vi "d1000 set pls outmode.vi"(10 "pls_outmode":i16, 11 "axis":i16) -> (3 "function return":u32)   [LabVIEW 2019, in "Dmc1000.lvlib"]
doc: "DMC1000_API DWORD WINAPI d1000_set_pls_outmode(short axis,short pls_outmode);"
uses:
  Dmc1000.lvlib
  Dmc1000.dll
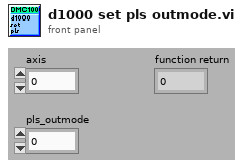
[diagram p1: front panel]
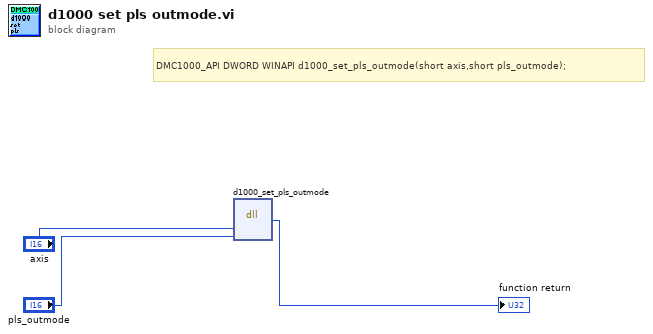
[diagram p0: block diagram]
diagram:
  # "DMC1000_API DWORD WINAPI d1000_set_pls_outmode(short axis,short pls_outmode);"
  n1 = dll-call lib="C:/Users/VIC/Desktop/Standar Program/System/LLB/DMC1000B/Dmc1000.*" fn="d1000_set_pls_outmode"("axis"="axis", "pls_outmode"="pls_outmode") -> (→"function return":u32)  [unwired: 5 in, 2 out]
